vi "顺序执行.vi"() -> ()   [LabVIEW 2021]
doc: "本VI是为《我和LabVIEW》一书编写的示例。\n关于本书的介绍请参考网页：\nhttp://ruanqizhen.spaces.live.com/blog/cns!5852D4F797C53FB6!4310.entry"
panel:
  in  "error in":errorcluster
  out "error out":errorcluster
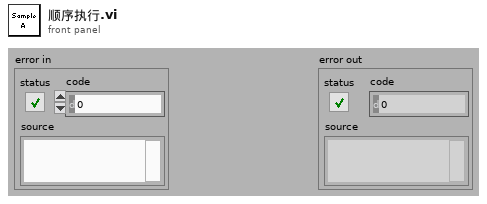
[diagram p1: front panel]
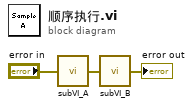
[diagram p0: block diagram]
diagram:
  n1 = call "subVI_A.vi"("error in (no error)"="error in") -> ("error out"=w2:errorcluster)
  n2 = call "subVI_B.vi"("error in (no error)"=w2) -> ("error out"=→"error out":errorcluster)
